vi "To Variant.vi"(8 "error in (no error)":errorcluster, 11 "Abs_Boolean_1D in":refnum<class "Abs_Boolean_1D.lvclass">) -> (0 "error out":errorcluster, 2 "Variant":variant, 3 "Abs_Boolean_1D out":refnum<class "Abs_Boolean_1D.lvclass">)   [LabVIEW 2021, in "Abs_Boolean_1D.lvclass"]
uses:
  Abs_Boolean_1D.lvclass
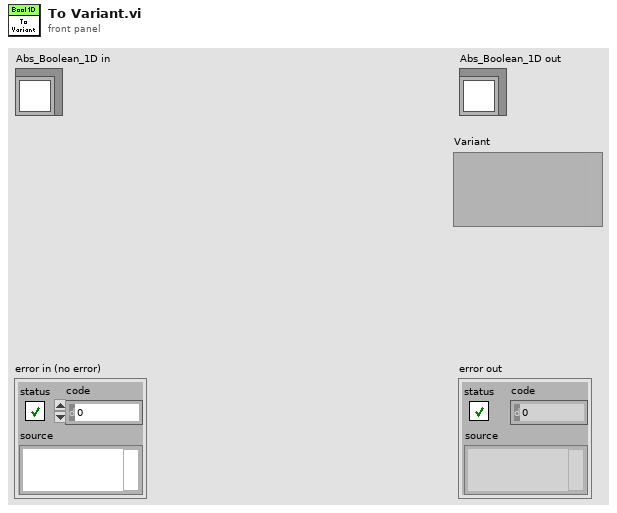
[diagram p1: front panel]
types:
  T1 = typedef "Abs_Boolean_1D.lvclass/Element Type.ctl" = bool
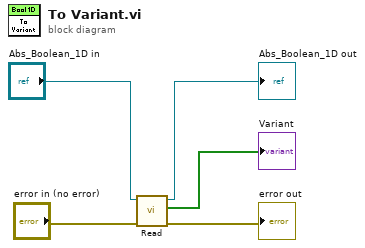
[diagram p0: block diagram]
diagram:
  n1 = call-dynamic "Read.vi"("error in (no error)"="error in (no error)", "Boolean in"="Abs_Boolean_1D in") -> ("error out"=→"error out":errorcluster, "Boolean 1D"=→"Variant":T1[], "Boolean out"=→"Abs_Boolean_1D out":refnum<class "Abs_Boolean_1D.lvclass">)  [unwired: 7 in]
